vi "LoggerRefnum Compare.vi"(1 "LoggerRef A":T1, 2 "LoggerRef B":T1) -> (5 "A=B?":bool)   [LabVIEW 2014]
uses:
  LoggerRef.ctl
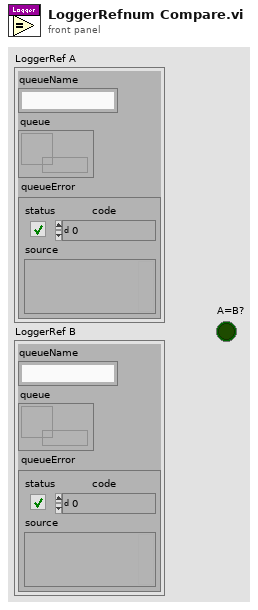
[diagram p1: front panel]
types:
  T1 = typedef "LoggerRef.ctl" = cluster{"queueName":string, "queue":refnum<queue>, "queueError":errorcluster}
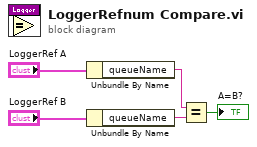
[diagram p0: block diagram]
diagram:
  n1 = Unbundle By Name("LoggerRef A") -> ("queueName"=w3:string)
  n2 = Unbundle By Name("LoggerRef B") -> ("queueName"=w2:string)
  n3 = Equal?(x=w3, y=w2) -> (x = y?=→"A=B?":bool)
